vi "Example_HTTPClient.vi"() -> ()   [LabVIEW 2018, in "HttpExamples.lvlib"]
doc: "<b> </b> <b> </b>\nHttpClient_NET\nJustin Young - Viviota\nCopyright (c) 2021\nLicense: BSD"
uses:
  HttpExamples.lvlib
  REST Client_NET/REST Client_NET.lvclass
  C:/Program Files (x86)/National Instruments/LabVIEW 2018/vi.lib/addons/_JKI.lib/REST Client/classes/REST Client/REST Client.lvclass
  <vilib>/addons/_JKI.lib/REST Client/classes/REST Client_JKI/REST Client_JKI.lvclass
  <vilib>/addons/_JKI.lib/REST Client/classes/REST Client/REST Client.lvclass
  <vilib>/addons/_JKI.lib/REST Client/classes/Response Headers/Response Headers.lvclass
panel:
  out "Error":errorcluster[](array[cluster])
  out "Response":string[](array[string])
  out "Values":string[][](array[string])
  out "Names":string[][](array[string])
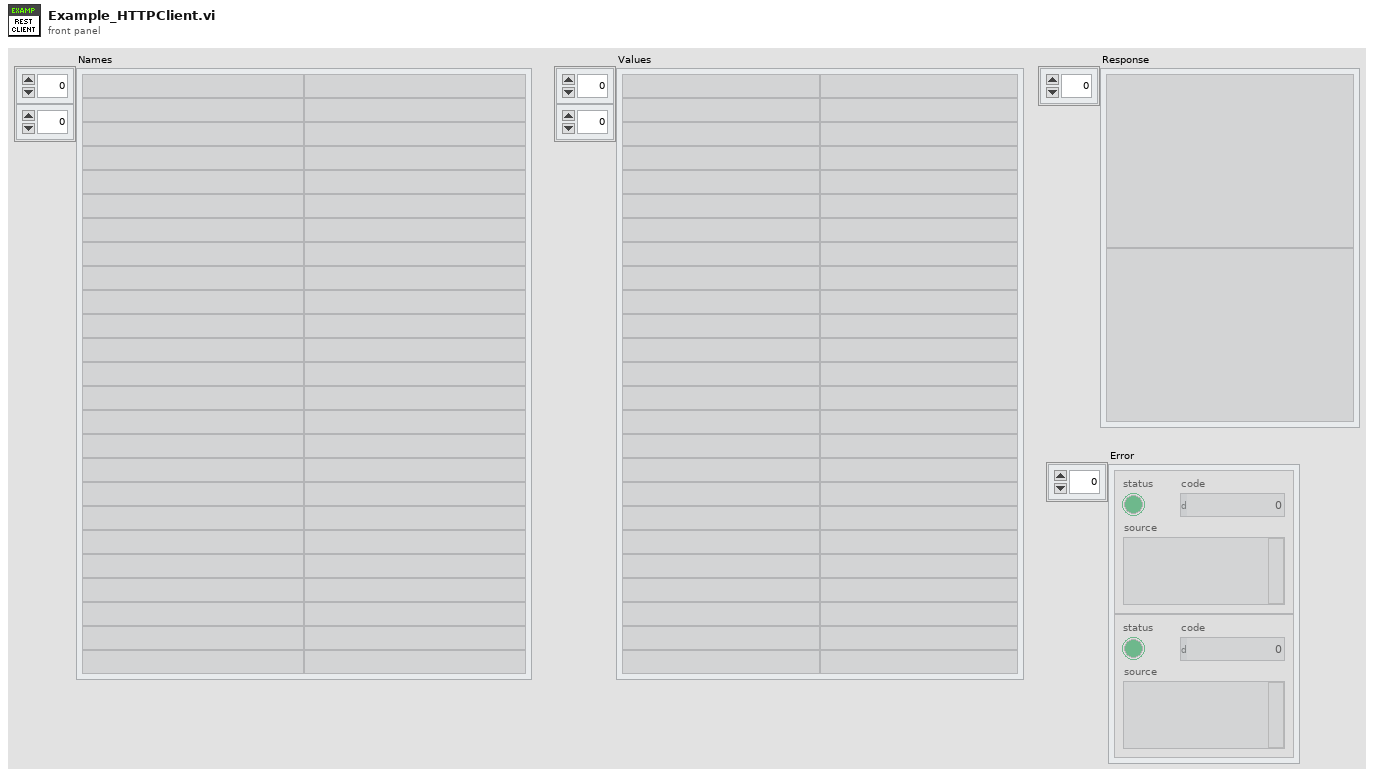
[diagram p1: front panel]
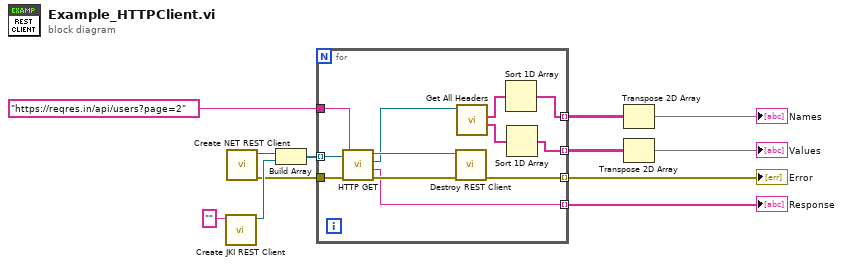
[diagram p0: block diagram]
diagram:
  n1 = call <vilib>:"Create JKI REST Client.vi"("Base URL"="") -> ("REST Client out"=w11:refnum<class "REST Client_JKI.lvclass">)  [unwired: 9 in, 1 out]
  n2 = call "Create NET REST Client.vi"() -> ("error out"=w9:errorcluster, "REST Client_NET out"=w12:refnum<class "REST Client_NET.lvclass">)  [unwired: 10 in]
  n3 = Build Array(w12, w11) -> (w10:refnum<class "REST Client.lvclass">[])
  n4 = for {
    tunnel: w10 -> [w21] mode=indexing
    tunnel: w9 -> [w20]
    tunnel: "https://reqres.in/api/users?page=2" ("Base URL") -> [w19]
    tunnel: [w18] -> w5 mode=indexing
    tunnel: [w16] -> w7 mode=indexing
    tunnel: [w13] -> w6 mode=indexing
    tunnel: [w17] -> w4 mode=indexing
    n5 = call-dynamic "HTTP GET.vi"("error in (no error)"=w20, "Path"=w19, "REST Client in"=w21) -> ("error out"=w23:errorcluster, "Response body"=w18:string, "Response Headers"=w22:refnum<class "Response Headers.lvclass">, "REST Client out"=w24:refnum<class "REST Client.lvclass">)  [unwired: 3 in, 2 out]
    n6 = call-dynamic "Destroy REST Client.vi"("error in (no error)"=w23, "REST Client in"=w24) -> ("error out"=w17:errorcluster)  [unwired: 9 in]
    n7 = call-dynamic "Get All Headers.vi"("Response Headers in"=w22) -> ("Values"=w14:string[], "Names"=w15:string[])  [unwired: 7 in, 2 out]
    n8 = Sort 1D Array(array=w15) -> (sorted array=w16:string[])
    n9 = Sort 1D Array(array=w14) -> (sorted array=w13:string[])
  }
  "Response" <- w5
  "Error" <- w4
  n10 = Transpose 2D Array(2D array=w7) -> (transposed array=→"Names":string[][])
  n11 = Transpose 2D Array(2D array=w6) -> (transposed array=→"Values":string[][])
